vi "Test.vi"() -> ()   [LabVIEW 2019]
panel:
  in  "Initial Capacity  (mAh) in":dbl=2500.0 format="%#_13g"
  out "Numeric":i32
  out "Waveform Graph":dbl[](graph)
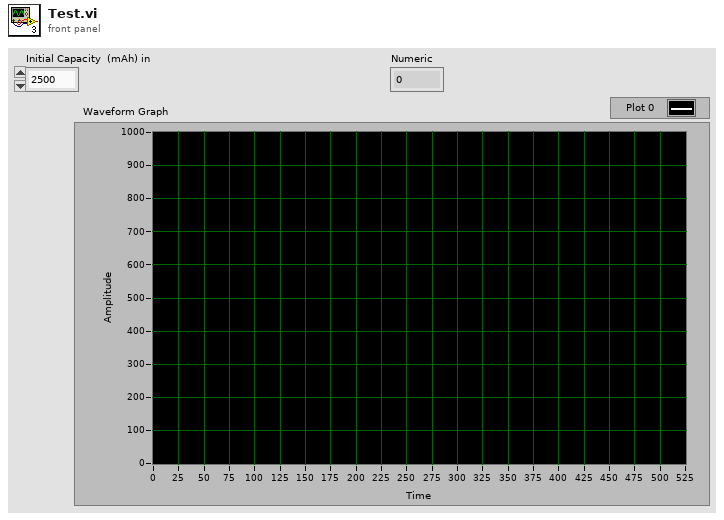
[diagram p1: front panel]
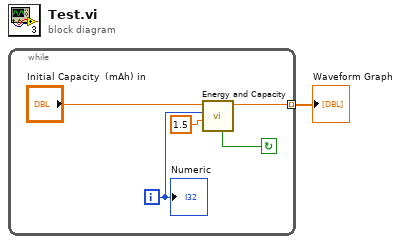
[diagram p0: block diagram]
diagram:
  n1 = while {
    tunnel: [w6] -> w1 mode=indexing
    i -> [w4]
    stop <- w2 continue-if-true
    n2 = call "Energy and Capacity.vi"("Voltage"=1.5, "Cycle"=w4, "Initial Capacity  (mAh) in"="Initial Capacity  (mAh) in") -> ("Capacity  (mAh)"=w6:dbl, "Pass"=w2:bool)  [unwired: 4 in, 3 out]
    "Numeric" <- w4
  }
  "Waveform Graph" <- w1
